vi "PostBuild.vi"(8 "error in (no error)":errorcluster, 9 "GeneratedFiles in":path[](array[path]), 10 "GeneratedDirectories in":path[](array[path]), 11 "Build in":refnum<class "AB_Targetfile.lvclass">) -> (0 "error out":errorcluster, 1 "GeneratedFiles out":path[](array[path]), 2 "GeneratedDirectories out":path[](array[path]), 3 "Build out":refnum<class "AB_Targetfile.lvclass">)   [LabVIEW 2020, in "AB_Targetfile.lvclass"]
uses:
  <vilib>/AppBuilder/AB_Classes/TargetFile/AB_Targetfile.lvclass
  e:/builds/penguin/labview/branches/2020/dev/dist/vi.lib/AppBuilder/AB_Classes/Build/AB_Build.lvclass
  <vilib>/AppBuilder/AB_Classes/Build/AB_Build.lvclass
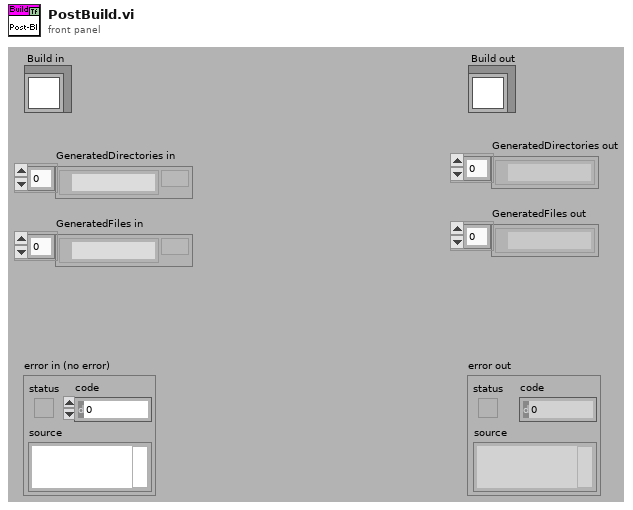
[diagram p1: front panel]
types:
  T1 = typedef "AB_Build.ctl" = cluster{"buildSpecName":string, "buildSpecDescription":string, "destinations":refnum<class "AB_Destination.lvclass">[], "exclusionOption":T2, "defaultLanguage":string, "supportedLanguages":string[], "excludedDirectories":path[], "buildContext":refnum<vi>, "buildObject":T3, "preview":bool, "programatic":bool, "progressBarEvents":T4, "userLog_Path":path, "preActionID":string, "preAction_Path":path, "postActionID":string, "postAction_Path":path, "eng_checkForBrokenVIs?":bool, "eng_verboseLinkerErrors?":bool, "localDest_Path":path, "targetDest_Path":path, "removeVIObject":u16, "cache":refnum<class "PreviewCache.lvclass">, "use cache":bool, "previewCache_ID":string, "buildCache_ID":string, "eng_TempLocalDest_Path":path, "eng_collectDependencies?":bool, "versionInfo":cluster{"buildVersion":cluster{"major":u16, "minor":u16, "patch":u16, "build":u16}, "autoIncrement":bool}, "eng_enableVIChecksums":bool}
  T2 = typedef "AB_Exclusion_Option.ctl" = cluster{"typedefs":bool, "polymorphicVIs":bool, "unusedLibraryItems":bool, "modifyLibraryFile":bool, "edit-timeDependencies":bool, "inlineVIs":bool, "dependent PPLs":bool, "dependent DLLs":bool}
  T3 = typedef "ItemRef.ctl" = u64
  T4 = typedef "provcom_ProgressBar_Events.ctl" = cluster{"newJob":refnum<user-event>, "newItem":refnum<user-event>, "errorMsg":T5, "cancel":refnum<user-event>}
  T5 = typedef "mxLvBuildError.ctl" = refnum<user-event>
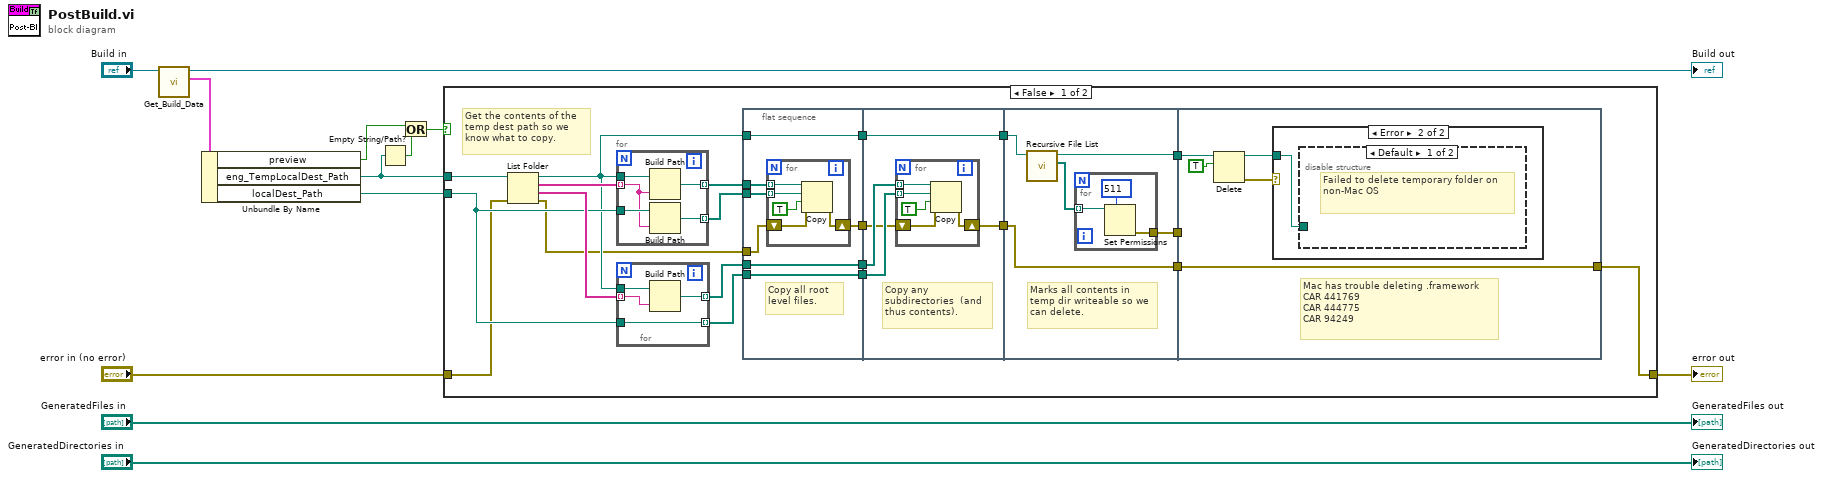
[diagram p0: block diagram]
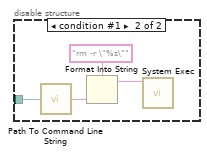
[diagram p3: hidden frame]
diagram:
  n1 = call <vilib>:"Get_Build_Data.vi"("Class in"="Build in") -> ("data"=w9:T1, "Class out"=→"Build out":refnum<class "AB_Targetfile.lvclass">)  [unwired: 1 in, 8 out]
  n2 = Unbundle By Name(w9) -> ("preview"=w5:bool, "eng_TempLocalDest_Path"=w8:path, "localDest_Path"=w7:path)
  n3 = Empty String/Path?(string/path=w8) -> (empty?=w4:bool)
  n4 = Or(x=w5, y=w4) -> (x .or. y?=w6:bool)
  n5 = case shown="False" w6 {
    tunnel: w8 -> [w30 _]
    tunnel: w7 -> [w28 _]
    tunnel: "error in (no error)" -> [w13 w83]
    tunnel: [w14 w83] -> w3
    frame False {
      # "Get the contents of the temp dest path so we know what to copy."
      n6 = List Folder(path=w30, error in=w13) -> (path out=w22:path, filenames=w33:string[], folder names=w29:string[], error out=w18:errorcluster)  [unwired: 2 in]
      n7 = for {
        tunnel: w33 -> [w80] mode=indexing
        tunnel: w22 -> [w81]
        tunnel: w28 -> [w82]
        tunnel: [w79] -> w32 mode=indexing
        tunnel: [w78] -> w31 mode=indexing
        n8 = Build Path(base path=w81, name or relative path=w80) -> (appended path=w79:path)
        n9 = Build Path(base path=w82, name or relative path=w80) -> (appended path=w78:path)
      }
      n10 = for {
        tunnel: w29 -> [w36] mode=indexing
        tunnel: w22 -> [w37]
        tunnel: w28 -> [w34]
        tunnel: [w35] -> w27 mode=indexing
        tunnel: [w34] -> w25 mode=indexing
        n11 = Build Path(base path=w37, name or relative path=w36) -> (appended path=w35:path)
      }
      n12 = flat-sequence {
        tunnel: w32 -> [w44]
        tunnel: w31 -> [w43]
        tunnel: w27 -> [w42]
        tunnel: [w42] -> w26
        tunnel: w25 -> [w41]
        tunnel: [w41] -> w24
        tunnel: w22 -> [w40]
        tunnel: [w40] -> w21
        tunnel: w18 -> [w39]
        tunnel: [w38] -> w17
        tunnel: w26 -> [w54]
        tunnel: w24 -> [w53]
        tunnel: w21 -> [w52]
        tunnel: [w52] -> w20
        tunnel: w17 -> [w51]
        tunnel: [w50] -> w16
        tunnel: [w63] -> w23
        tunnel: w20 -> [w62]
        tunnel: [w61] -> w19
        tunnel: w16 -> [w60]
        tunnel: [w60] -> w15
        tunnel: w23 -> [w71]
        tunnel: w19 -> [_]
        tunnel: w15 -> [w70]
        tunnel: [w70] -> w14
        frame #0 {
          # "Copy all root level files."
          n13 = for {
            tunnel: w44 -> [w49] mode=indexing
            tunnel: w43 -> [w48] mode=indexing
            shift-right: [w45] -> w38
            shift-left: w39 -> [w46]
            n14 = Copy(8:w46, 9:TRUE ("overwrite (F)"), 10:w48, 11:w49) -> (0:w45:errorcluster)  [unwired: 1 in, 2 out]
          }
        }
        frame #1 {
          # "Copy any subdirectories  (and thus contents)."
          n15 = for {
            tunnel: w54 -> [w59] mode=indexing
            tunnel: w53 -> [w58] mode=indexing
            shift-right: [w55] -> w50
            shift-left: w51 -> [w56]
            n16 = Copy(8:w56, 9:TRUE ("overwrite (F)"), 10:w58, 11:w59) -> (0:w55:errorcluster)  [unwired: 1 in, 2 out]
          }
        }
        frame #2 {
          # "Marks all contents in temp dir writeable so we can delete."
          n17 = call <vilib>:"Recursive File List.vi"("Folder Path"=w62) -> ("All Files in Dir"=w64:path[], "dup Folder Path"=w63:path)  [unwired: 2 in, 7 out]
          n18 = for {
            tunnel: w64 -> [w66] mode=indexing
            tunnel: [w65] -> w61
            n19 = Set Permissions(7:i16 511 ("permissions"), 11:w66) -> (0:w65:errorcluster)  [unwired: 1 in, 3 out]
          }
        }
        frame #3 {
          # "Mac has trouble deleting .framework\nCAR 441769\nCAR 444775\nCAR 94249"
          n20 = Delete(path (use dialog)=w71, entire hierarchy (F)=TRUE) -> (deleted path=w68:path, error out=w69:errorcluster)  [unwired: 1 in, 3 out]
          n21 = case shown="Error" w69 {
            tunnel: w68 -> [_ w73]
            frame No Error {
            }
            frame Error {
              n22 = disable-structure shown="Default" {
                disable-tunnel: w73 -> [_ w75]
                frame condition #0 (active) {
                  # "Failed to delete temporary folder on non-Mac OS"
                }
                frame condition #1 {
                  n23 = call <vilib>:"Path To Command Line String.vi"("path"=w75) -> ("string"=w74:string)
                  n24 = Format Into String(format string="rm -r \"%s\"", w74) -> (resulting string=w76:string)  [unwired: 2 in, 1 out]
                  n25 = call <vilib>:"System Exec.vi"("command line"=w76) -> ()  [unwired: 7 in, 4 out]
                }
              }
            }
          }
        }
      }
    }
    frame True {
    }
  }
  "error out" <- w3
  "GeneratedDirectories out" <- "GeneratedDirectories in"
  "GeneratedFiles out" <- "GeneratedFiles in"
